vi "trigger-test.vi"() -> ()   [LabVIEW 2020]
uses:
  <instrlib>/niDMM/nidmm.llb/niDMM Waveform Function.ctl
  <instrlib>/niDMM/nidmm.llb/niDMM Trigger.ctl
  <vilib>/DAQmx/create/channels.llb/DAQmx Create Channel (CO-Pulse Generation-Frequency).vi
  <vilib>/DAQmx/configure/timing.llb/DAQmx Timing (Implicit).vi
  <instrlib>/niDMM/nidmm.llb/niDMM Fetch Waveform (waveform data).vi
panel:
  in  "Trigger Source":T1=enum."TTL 0"
  in  "Function":T2=1003 items=["Waveform_Voltage"=1003, "Waveform_Current"=1004]
  in  "Device Name":refnum<k15>="NI_DMM"
  out "Waveform Graph":dynamicdata(graph)
  in  "counter output":tag="NI_Timing/ctr0"
  out "error out":errorcluster
  in  "source terminal":tag="/NI_Timing/PFI39"
  in  "destination terminal":tag="/NI_AnaIn1/PXI_Trig0"
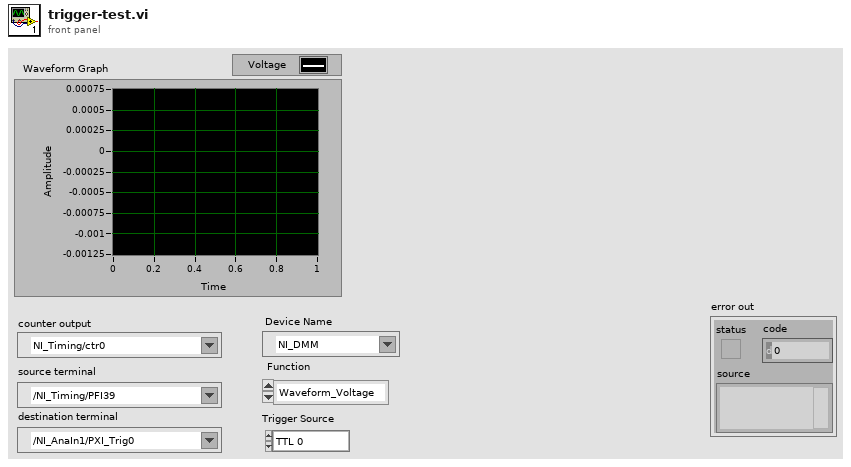
[diagram p1: front panel]
types:
  T1 = typedef "niDMM Trigger.ctl" = enum16{"Immediate", "External", "TTL 0", "TTL 1", "TTL 2", "TTL 3", "TTL 4", "TTL 5", "TTL 6", "Software", "TTL 7", "PXI Star", "LBR Trig 1", "Aux Trig 1"}
  T2 = typedef "niDMM Waveform Function.ctl" = i32
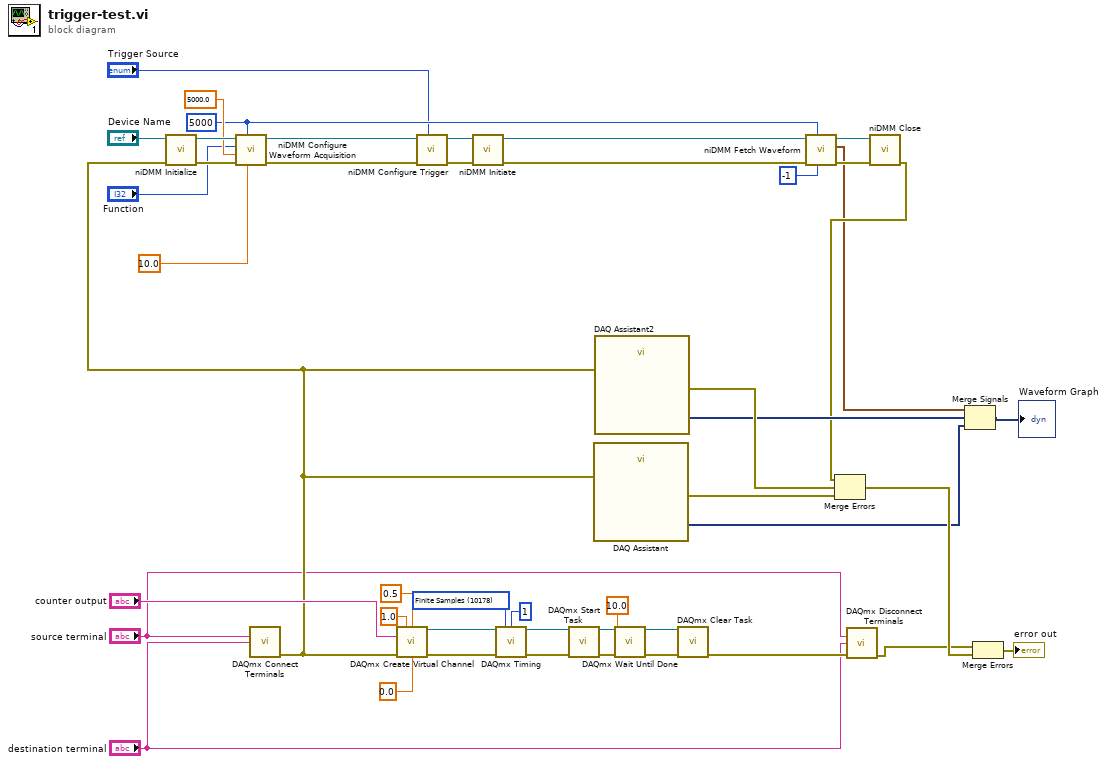
[diagram p0: block diagram]
diagram:
  w6 = 10178 items=["Finite Samples"=10178, "Continuous Samples"=10123, "Hardware Timed Single Point"=12522] ("sample mode")
  w32 = 5000 ("Number of samples")
  n1 = call <vilib>:"DAQmx Connect Terminals.vi"("source terminal"="source terminal", "destination terminal"="destination terminal") -> ("error out"=w21:errorcluster)  [unwired: 13 in]
  n2 = call <instrlib>:"niDMM Initialize.vi"("error in (no error)"=w21, "Instrument Descriptor"="Device Name") -> ("error out"=w37:errorcluster, "instrument handle out"=w38:refnum<k15>)  [unwired: 8 in]
  n3 = call <instrlib>:"niDMM Configure Waveform Acquisition.vi"("Range"=10.0, "Waveform Points"=w32, "error in (no error)"=w37, "Rate"=5000.0 ("Sample Rate"), "Function"="Function", "instrument handle"=w38) -> ("error out"=w20:errorcluster, "instrument handle out"=w27:refnum<k15>)  [unwired: 4 in]
  n4 = call-poly <vilib>:"DAQmx Create Virtual Channel.vi"("frequency"=1.0, "duty cycle"=0.5, "counter"="counter output", "error in"=w21, "initial delay"=0.0) -> ("task out"=w4:refnum<k21>, "error out"=w5:errorcluster)  [unwired: 9 in]
  n5 = call <instrlib>:"niDMM Configure Trigger.vi"("Trigger Source"="Trigger Source", "error in (no error)"=w20, "instrument handle"=w27) -> ("error out"=w29:errorcluster, "instrument handle out"=w30:refnum<k15>)  [unwired: 7 in]
  n6 = call <instrlib>:"niDMM Initiate.vi"("error in (no error)"=w29, "instrument handle"=w30) -> ("error out"=w25:errorcluster, "instrument handle out"=w26:refnum<k15>)  [unwired: 8 in]
  n7 = call-poly <vilib>:"DAQmx Timing.vi"("task/channels in"=w4, "sample mode"=w6, "samples per channel"=1, "error in"=w5) -> ("task out"=w14:refnum<k21>, "error out"=w15:errorcluster)  [unwired: 10 in]
  n8 = call <vilib>:"DAQmx Start Task.vi"("task/channels in"=w14, "error in"=w15) -> ("task out"=w12:refnum<k21>, "error out"=w13:errorcluster)  [unwired: 12 in]
  n9 = call "DAQ Assistant"("error in"=w21) -> ("data"=w40:dynamicdata, "error out"=w44:errorcluster)  [unwired: 16 in, 1 out]
  n10 = call "DAQ Assistant2"("error in"=w21) -> ("data"=w41:dynamicdata, "error out"=w43:errorcluster)  [unwired: 16 in, 1 out]
  n11 = call <vilib>:"DAQmx Wait Until Done.vi"("task/channels in"=w12, "timeout (sec)"=10.0, "error in"=w13) -> ("task out"=w16:refnum<k21>, "error out"=w17:errorcluster)  [unwired: 11 in]
  n12 = call <vilib>:"DAQmx Clear Task.vi"("task in"=w16, "error in"=w17) -> ("error out"=w18:errorcluster)  [unwired: 13 in]
  n13 = call-poly <instrlib>:"niDMM Fetch Waveform.vi"("Maximum Time (msec)"=-1, "Number To Fetch"=w32, "error in (no error)"=w25, "instrument handle"=w26) -> ("error out"=w28:errorcluster, "Waveform Data"=w22:waveform(dbl), "instrument handle out"=w31:refnum<k15>)  [unwired: 4 in, 1 out]
  n14 = call <vilib>:"DAQmx Disconnect Terminals.vi"("source terminal"="source terminal", "destination terminal"="destination terminal", "error in"=w18) -> ("error out"=w19:errorcluster)  [unwired: 12 in]
  n15 = call <instrlib>:"niDMM Close.vi"("error in (no error)"=w28, "instrument handle"=w31) -> ("error out"=w23:errorcluster)  [unwired: 9 in]
  n16 = Merge Errors(w23, w43, w44) -> (w42:errorcluster)
  n17 = Merge Signals(w22, w41, w40) -> (→"Waveform Graph":dynamicdata)
  n18 = Merge Errors(w19, w42) -> (→"error out":errorcluster)
